vi "Get DTC References.vi"(8 "error in (no error)":errorcluster, 10 "DM GUID":string, 11 "Item Ref in":T1 format="%.0x") -> (0 "error out":errorcluster, 1 "Data":T1[](array[typedef]) format="%.0x", 2 "Active":T1[](array[typedef]) format="%.0x", 3 "Section Ref out":T1 format="%.0x")   [LabVIEW 2019, in "J1939 Addon System Explorer.lvlib"]
uses:
  J1939 Addon System Explorer.lvlib
  <vilib>/NI VeriStand/Custom Device API/Custom Device Item Ref.ctl
  Addon Shared/SubVIs/Constants.vi
  <vilib>/NI VeriStand/Custom Device Tools/Custom Device Utility Library/NI VeriStand - Search for Item by GUID.vi
  <vilib>/NI VeriStand/Custom Device Tools/Custom Device Utility Library/NI VeriStand - Search for Item by Name.vi
  <vilib>/NI VeriStand/Custom Device Tools/Custom Device Utility Library/NI VeriStand - Search for All Items by GUID.vi
  <vilib>/NI VeriStand/Custom Device Tools/Custom Device Utility Library/Custom Device Utility Library.lvlib
  Addon Shared/J1939 Addon Shared.lvlib
  <vilib>/NI VeriStand/Custom Device API/Custom Device API.lvlib
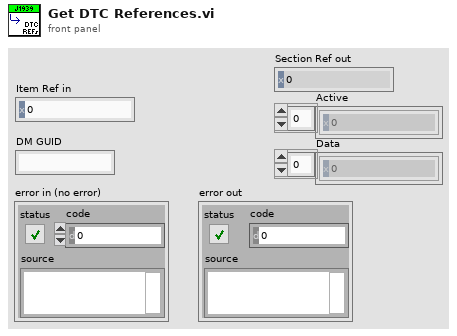
[diagram p1: front panel]
types:
  T1 = typedef "Custom Device API.lvlib/Custom Device Item Ref.ctl" = u64
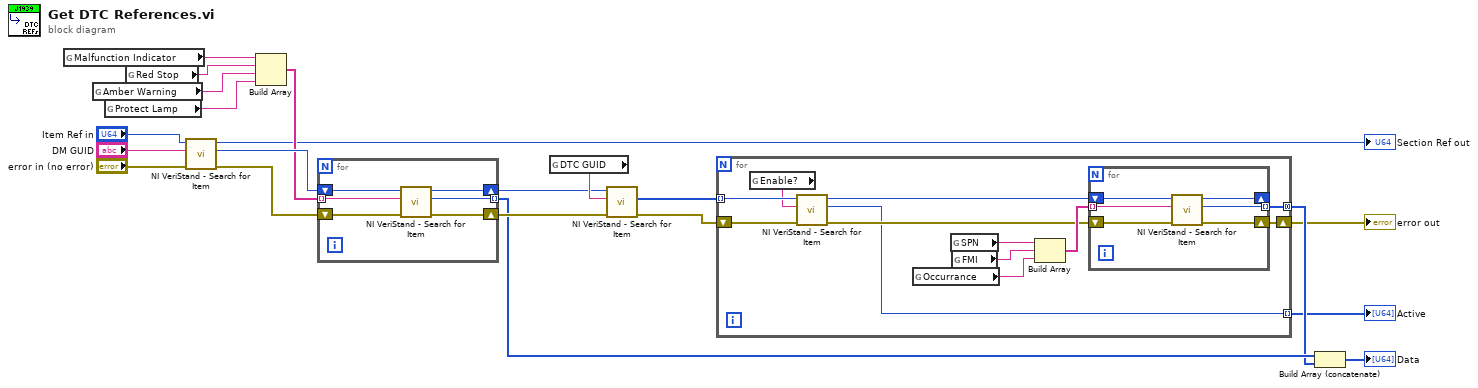
[diagram p0: block diagram]
diagram:
  n1 = global read "Constants.vi" "Malfunction Indicator"() -> (w11:string)
  n2 = global read "Constants.vi" "Amber Warning"() -> (w13:string)
  n3 = global read "Constants.vi" "Protect Lamp"() -> (w14:string)
  n4 = global read "Constants.vi" "Red Stop"() -> (w12:string)
  n5 = call-poly <vilib>:"NI VeriStand - Search for Item.vi"("error in"="error in (no error)", "Item GUID"="DM GUID", "Section Ref in"="Item Ref in") -> ("error out"=w10:errorcluster, "Item Ref"=w17:T1, "Section Ref out"=→"Section Ref out":T1)  [unwired: 5 in, 1 out]
  n6 = Build Array(w11, w12, w13, w14) -> (w15:string[])
  n7 = for {
    shift-right: [w25] -> w16
    shift-left: w10 -> [w26]
    tunnel: w15 -> [w24] mode=indexing
    tunnel: [w23] -> w5 mode=indexing
    shift-right: [w22] -> w18
    shift-left: w17 -> [w27]
    n8 = call-poly <vilib>:"NI VeriStand - Search for Item.vi"("error in"=w26, "Item Name"=w24, "Section Ref in"=w27) -> ("error out"=w25:errorcluster, "Item Ref"=w23:T1, "Section Ref out"=w22:T1)  [unwired: 5 in, 1 out]
  }
  n9 = global read "Constants.vi" "DTC GUID"() -> (w19:string)
  n10 = call-poly <vilib>:"NI VeriStand - Search for Item.vi"("error in"=w16, "Item GUID"=w19, "Section Ref in"=w18) -> ("error out"=w20:errorcluster, "Item Refs"=w21:T1[])  [unwired: 5 in, 2 out]
  n11 = for {
    tunnel: w21 -> [w34] mode=indexing
    shift-right: [w39] -> w3
    shift-left: w20 -> [w32]
    tunnel: [w29] -> w2 mode=indexing
    tunnel: [w28] -> w4 mode=concatenating
    n12 = global read "Constants.vi" "Enable?"() -> (w30:string)
    n13 = call-poly <vilib>:"NI VeriStand - Search for Item.vi"("error in"=w32, "Item Name"=w30, "Section Ref in"=w34) -> ("error out"=w31:errorcluster, "Item Ref"=w29:T1, "Section Ref out"=w33:T1)  [unwired: 5 in, 1 out]
    n14 = global read "Constants.vi" "Occurrance"() -> (w36:string)
    n15 = global read "Constants.vi" "SPN"() -> (w38:string)
    n16 = global read "Constants.vi" "FMI"() -> (w37:string)
    n17 = Build Array(w38, w37, w36) -> (w35:string[])
    n18 = for {
      shift-right: [w43] -> w39
      shift-left: w31 -> [w44]
      tunnel: w35 -> [w42] mode=indexing
      tunnel: [w41] -> w28 mode=indexing
      shift-right: [w40] -> _
      shift-left: w33 -> [w45]
      n19 = call-poly <vilib>:"NI VeriStand - Search for Item.vi"("error in"=w44, "Item Name"=w42, "Section Ref in"=w45) -> ("error out"=w43:errorcluster, "Item Ref"=w41:T1, "Section Ref out"=w40:T1)  [unwired: 5 in, 1 out]
    }
  }
  "error out" <- w3
  "Active" <- w2
  n20 = Build Array (concatenate)(w5, w4) -> (→"Data":T1[])
